vi "Recipe_u_1.vi"() -> ()   [LabVIEW 2011]
uses:
  Globals/Global VI.vi
  <vilib>/Utility/file.llb/Read From Spreadsheet File (string).vi
panel:
  in  "Recipe":i32(listbox)
  in  "Save As Button":bool
  in  "Save Button":bool
  in  "Open Button":bool
  in  "New Button":bool
  # "Recipe"
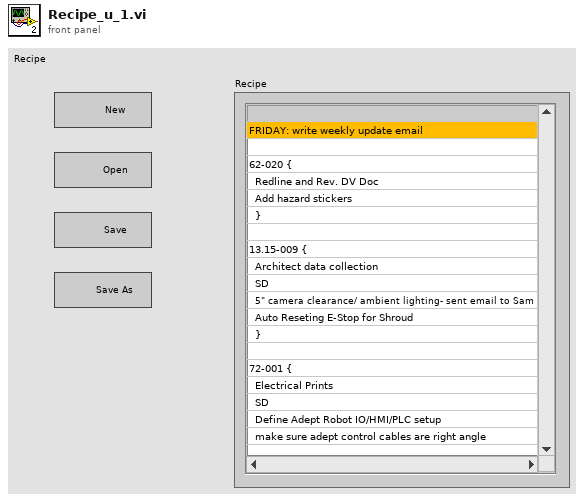
[diagram p1: front panel]
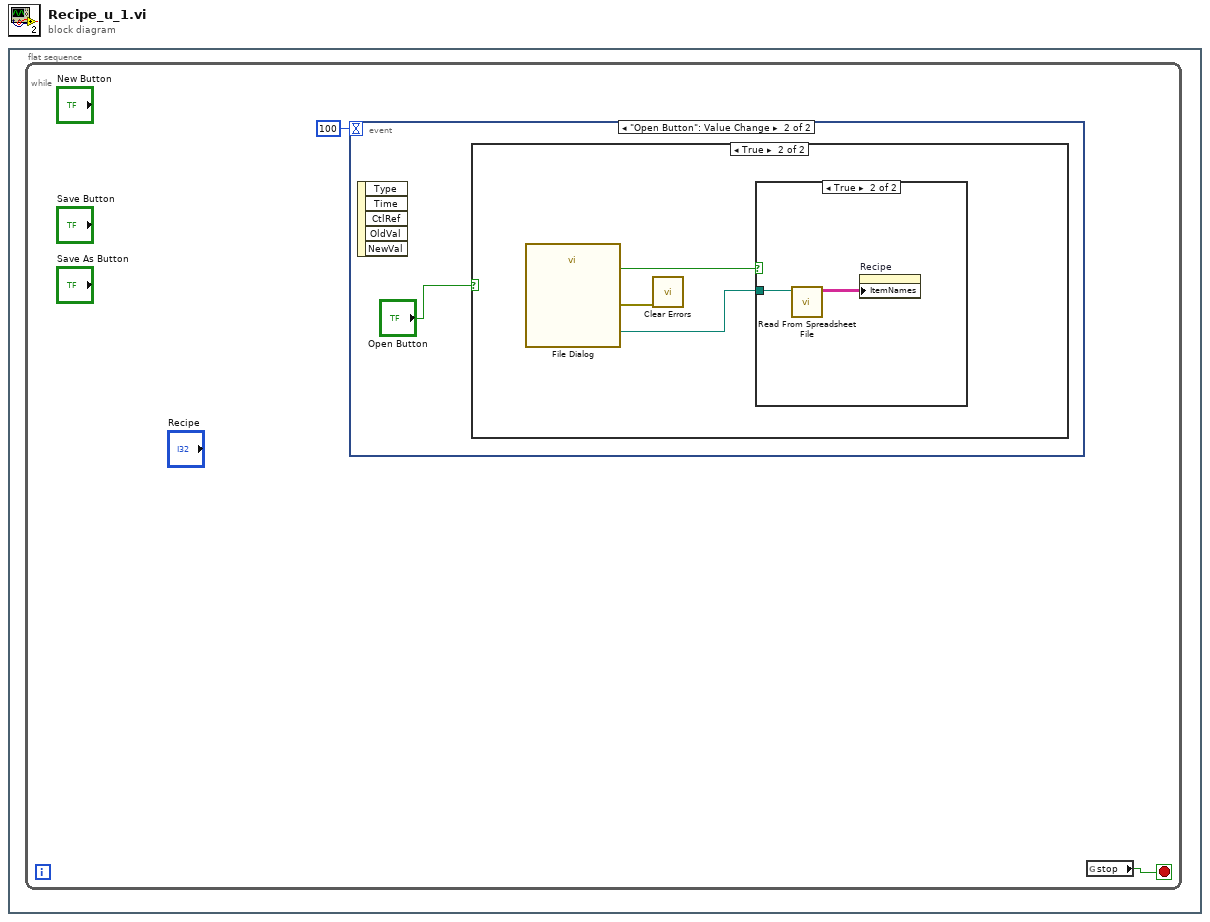
[diagram p0: block diagram]
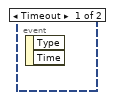
[diagram p2: hidden frame]
diagram:
  n1 = flat-sequence {
    frame #0 {
      n2 = while {
        stop <- w2 stop-if-true
        n3 = event shown="[1] \"Open Button\": Value Change" {
          selector: _ -> [_ _]
          dyn-events: _ -> [_ _]
          timeout: 100 -> [_ _]
          event Timeout {
            n4 = event-data() -> ()  [unwired: 1 in, 2 out]
          }
          event "Open Button": Value Change {
            n5 = event-data() -> ()  [unwired: 1 in, 5 out]
            n6 = case shown="True" "Open Button" {
              frame False {
              }
              frame True {
                n7 = call "File Dialog"() -> ("selected path"=w6:path, "exists"=w5:bool, "error out"=w4:errorcluster)  [unwired: 12 in, 1 out]
                n8 = call <vilib>:"Clear Errors.vi"("error in (no error)"=w4) -> ()  [unwired: 6 in, 1 out]
                n9 = case shown="True" w5 {
                  tunnel: w6 -> [_ w7]
                  frame False {
                  }
                  frame True {
                    n10 = call-poly <vilib>:"Read From Spreadsheet File.vi"("file path (dialog if empty)"=w7) -> ("all rows"=w8:string[][])  [unwired: 6 in, 4 out]
                    n11 = property on="Recipe" class="MCListbox (strict)"("ItemNames"=w8) -> ()  [unwired: 2 in, 2 out]
                  }
                }
              }
            }
          }
        }
        n12 = global read "Global VI.vi" "stop"() -> (w2:bool)
      }
    }
  }
